vi "Load cell setup.vi"(8 "error in (no error)":errorcluster) -> (0 "error out":errorcluster)   [LabVIEW 2016]
uses:
  Controls/Gain modes.ctl
  <vilib>/Utility/inputDevices.llb/keyboardAcquire.vi
  <vilib>/Utility/inputDevices.llb/closeKeyboard.vi
panel:
  in  "Offset":dbl
  in  "Gain":dbl=1.0
  in  "Confirm":bool
  in  "Cancel":bool
  # "TEST SETTINGS"
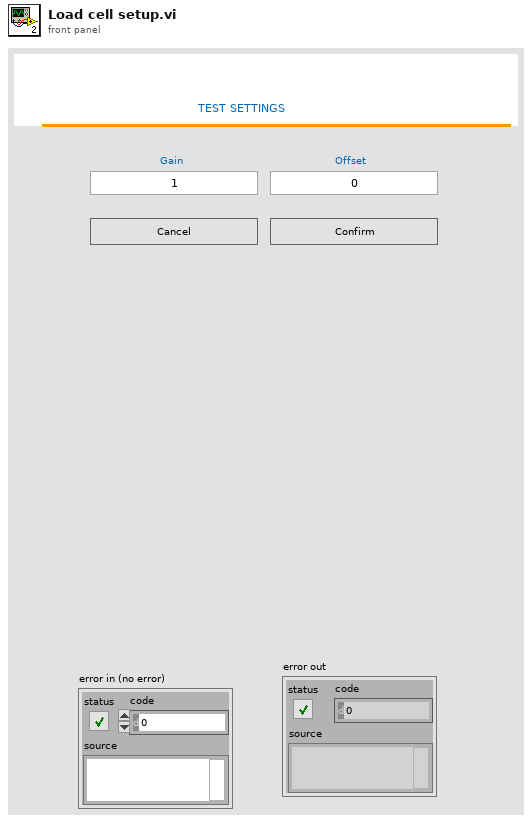
[diagram p1: front panel]
types:
  T1 = typedef "Gain modes.ctl" = enum16{"Initalise", "Get", "Set"}
  T2 = enum16{"0", "1", "2", "3", "4", "5", "6", "7", "8", "9", "A", "B", "C", "D", "E", "F", "G", "H", "I", "J", "K", "L", "M", "N", "O", "P", "Q", "R", "S", "T", "U", "V", "W", "X", "Y", "Z", "F1", "F2", "F3", "F4", "F5", "F6", "F7", "F8", "F9", "F10", "F11", "F12", "F13", "F14", "F15", "ADD", "BACK", "BACKSLASH", "CAPITAL", "COMMA", "DECIMAL", "DELETE", "DIVIDE", "DOWN", "END", "EQUALS", "ESCAPE", "GRAVE (`)", "HOME", "INSERT", "LBRACKET", "LCONTROL", "LEFT", "L ALT", "LSHIFT", "LWIN", "MINUS", "MULTIPLY", "NEXT", "NUMLOCK", "NUMPAD_0", "NUMPAD_1", "NUMPAD_2", "NUMPAD_3", "NUMPAD_4", "NUMPAD_5", "NUMPAD_6", "NUMPAD_7", "NUMPAD_8", "NUMPAD_9", "PAUSE", "PERIOD", "PRIOR (PG UP)", "RBRACKET", "RCONTROL", "RETURN", "RIGHT", "R ALT", "RSHIFT", "RWIN", "SCROLL", "SEMICOLON", "SLASH", "SPACE", "SUBTRACT", "TAB", "UP", "ENTER (num pad)", "' (quote)"}
  T3 = enum16{"0", "1", "2", "3", "4", "5", "6", "7", "8", "9", "A", "B", "C", "D", "E", "F", "G", "H", "I", "J", "K", "L", "M", "N", "O", "P", "Q", "R", "S", "T", "U", "V", "W", "X", "Y", "Z", "F1", "F2", "F3", "F4", "F5", "F6", "F7", "F8", "F9", "F10", "F11", "F12", "F13", "F14", "F15", "ADD", "BACK", "BACKSLASH", "CAPITAL", "COMMA", "DECIMAL", "DELETE", "DIVIDE", "DOWN", "END", "EQUALS", "ESCAPE", "GRAVE (`)", "HOME", "INSERT", "LBRACKET", "LCONTROL", "LEFT", "L ALT", "LSHIFT", "LWIN", "MINUS", "MULTIPLY", "NEXT", "NUMLOCK", "NUMPAD_0", "NUMPAD_1", "NUMPAD_2", "NUMPAD_3", "NUMPAD_4", "NUMPAD_5", "NUMPAD_6", "NUMPAD_7", "NUMPAD_8", "NUMPAD_9", "PAUSE", "PERIOD", "PRIOR (PG UP)", "RBRACKET", "RCONTROL", "RETURN", "RIGHT", "R ALT", "RSHIFT", "RWIN", "SCROLL", "SEMICOLON", "SLASH", "SPACE", "SUBTRACT", "TAB", "UP", "ENTER (num pad)", "' (quote)"}[]
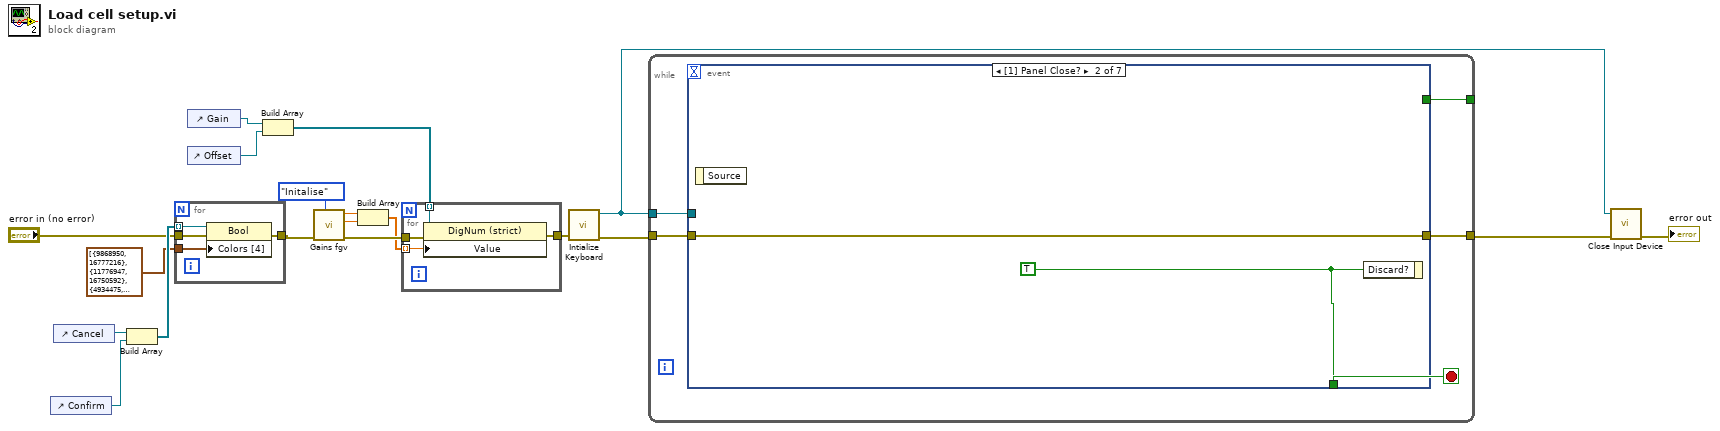
[diagram p0: block diagram]
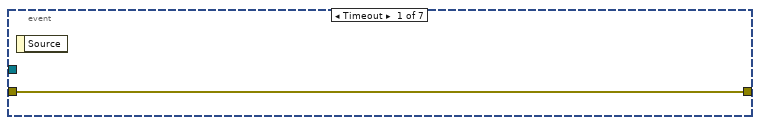
[diagram p2: hidden frame]
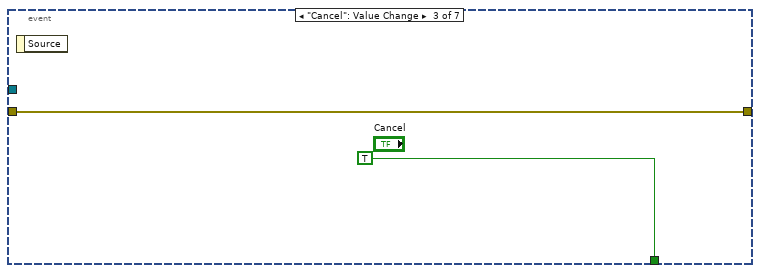
[diagram p3: hidden frame]
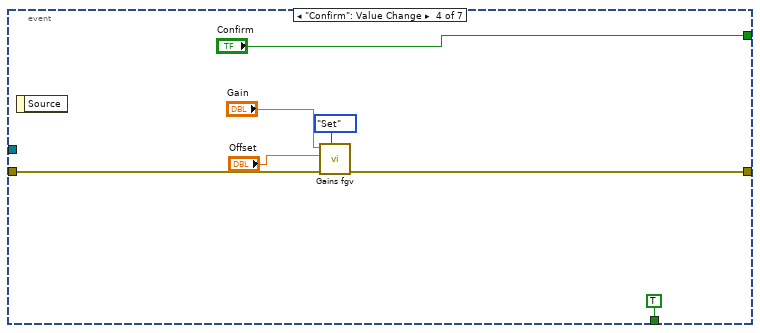
[diagram p4: hidden frame]
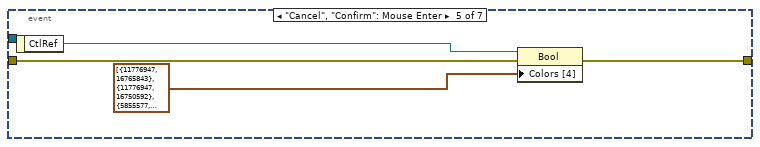
[diagram p5: hidden frame]
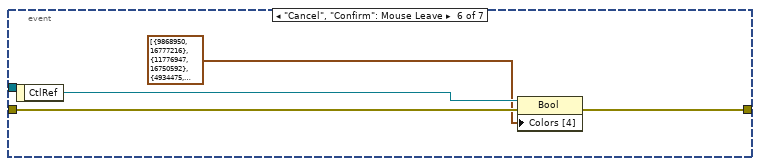
[diagram p6: hidden frame]
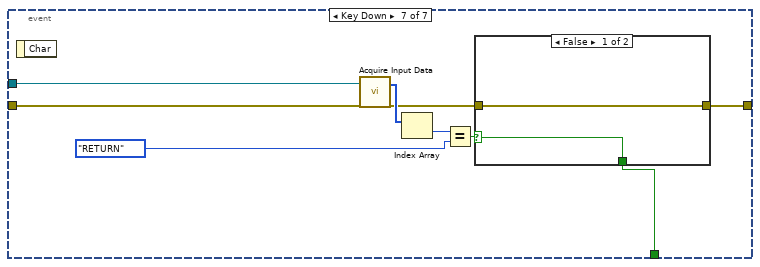
[diagram p7: hidden frame]
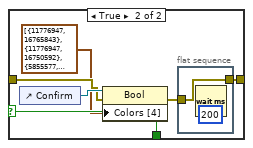
[diagram p8: hidden frame]
diagram:
  n1 = control-ref of="Confirm"() -> (w18:refnum<vi>)
  n2 = control-ref of="Cancel"() -> (w19:refnum<vi>)
  n3 = Build Array(w19, w18) -> (w17:refnum<vi>[])
  n4 = for {
    tunnel: "error in (no error)" -> [w23]
    tunnel: [w22] -> w10
    tunnel: w17 -> [w21] mode=indexing
    tunnel: cluster{u32, u32}[] [{9868950, 16777216}, {11776947, 16750592}, {4934475, 16777216}, {5855577, 8342528}] ("Colors [4]") -> [w20]
    n5 = property class="Bool"(reference=w21, error in=w23, "Colors [4]"=w20) -> (error out=w22:errorcluster)  [unwired: 1 out]
  }
  n6 = control-ref of="Gain"() -> (w4:refnum<vi>)
  n7 = control-ref of="Offset"() -> (w3:refnum<vi>)
  n8 = Build Array(w4, w3) -> (w1:refnum<vi>[])
  n9 = call "Gains fgv.vi"("Mode"=Gain_modes."Initalise", "error in (no error)"=w10) -> ("error out"=w8:errorcluster, "Offset"=w6:dbl, "Gain"=w7:dbl)  [unwired: 7 in]
  n10 = Build Array(w7, w6) -> (w5:dbl[])
  n11 = for {
    tunnel: w8 -> [w27]
    tunnel: w5 -> [w26] mode=indexing
    tunnel: w1 -> [w25] mode=indexing
    tunnel: [w24] -> w2
    n12 = property class="DigNum (strict)"(reference=w25, error in=w27, "Value"=w26) -> (error out=w24:errorcluster)  [unwired: 1 out]
  }
  n13 = call <vilib>:"Intialize Keyboard.vi"("error in (no error)"=w2) -> ("error out"=w15:errorcluster, "device ID"=w12:refnum<k1>)  [unwired: 9 in]
  n14 = while {
    tunnel: w15 -> [w31]
    tunnel: [w30] -> w13
    tunnel: w12 -> [w29]
    tunnel: [w28] -> _
    stop <- w32 stop-if-true
    n15 = event shown="[1] Panel Close?" {
      selector: _ -> [_ _ _ _ _ _ _]
      dyn-events: _ -> [_ _ _ _ _ _ _]
      timeout: _ -> [_ _ _ _ _ _ _]
      tunnel: [_ w35 TRUE ("Discard?") TRUE ("Discard?") _ _ w55] -> w32
      tunnel: w31 -> [w33 w34 w36 w43 w47 w52 w61]
      tunnel: [w33 w34 w36 w39 w46 w51 w53] -> w30
      tunnel: w29 -> [_ _ _ _ _ _ w60]
      tunnel: [_ _ _ "Confirm" _ _ _] -> w28
      event Timeout {
        n16 = event-data() -> ()  [unwired: 1 in, 1 out]
      }
      event Panel Close? {
        w35 = TRUE ("Discard?")
        n17 = event-data() -> ()  [unwired: 1 in, 1 out]
        n18 = event-data("Discard?"=w35) -> ()  [unwired: 1 in, 1 out]
      }
      event "Cancel": Value Change {
        n19 = event-data() -> ()  [unwired: 1 in, 1 out]
      }
      event "Confirm": Value Change {
        n20 = event-data() -> ()  [unwired: 1 in, 1 out]
        n21 = call "Gains fgv.vi"("Mode"=Gain_modes."Set", "error in (no error)"=w43, "Offset"="Offset", "Gain"="Gain") -> ("error out"=w39:errorcluster)  [unwired: 5 in, 2 out]
      }
      event "Cancel", "Confirm": Mouse Enter {
        n22 = event-data() -> ("CtlRef"=w45:refnum<vi>)  [unwired: 1 in]
        n23 = property class="Bool"(reference=w45, error in=w47, "Colors [4]"=cluster{u32, u32}[] [{11776947, 16765843}, {11776947, 16750592}, {5855577, 8350025}, {5855577, 8342528}]) -> (error out=w46:errorcluster)  [unwired: 1 out]
      }
      event "Cancel", "Confirm": Mouse Leave {
        n24 = event-data() -> ("CtlRef"=w50:refnum<vi>)  [unwired: 1 in]
        n25 = property class="Bool"(reference=w50, error in=w52, "Colors [4]"=cluster{u32, u32}[] [{9868950, 16777216}, {11776947, 16750592}, {4934475, 16777216}, {5855577, 8342528}]) -> (error out=w51:errorcluster)  [unwired: 1 out]
      }
      event Key Down {
        n26 = event-data() -> ()  [unwired: 1 in, 1 out]
        n27 = call-poly <vilib>:"Acquire Input Data.vi"("device ID"=w60, "error in (no error)"=w61) -> ("keys pressed"=w59:T3, "error out"=w54:errorcluster)  [unwired: 15 in, 1 out]
        n28 = Index Array(array=w59) -> (element=w58:T2)  [unwired: 1 in]
        n29 = Equal?(x=w58, y=T2."RETURN" ("keyType 3")) -> (x = y?=w56:bool)
        n30 = case shown="False" w56 {
          selector: w56 -> [w62 w69]
          tunnel: [w62 w69] -> w55
          tunnel: w54 -> [w63 w67]
          tunnel: [w63 w64] -> w53
          frame False {
          }
          frame True {
            n31 = control-ref of="Confirm"() -> (w68:refnum<vi>)
            n32 = property class="Bool"(reference=w68, error in=w67, "Colors [4]"=cluster{u32, u32}[] [{11776947, 16765843}, {11776947, 16750592}, {5855577, 8350025}, {5855577, 8342528}]) -> (error out=w65:errorcluster)  [unwired: 1 out]
            n33 = flat-sequence {
              tunnel: w65 -> [w70]
              tunnel: [w70] -> w64
              frame #0 {
                n34 = Wait (ms)(milliseconds to wait=u32 200) -> ()  [unwired: 1 out]
              }
            }
          }
        }
      }
    }
  }
  n35 = call-poly <vilib>:"Close Input Device.vi"("error in (no error)"=w13, "device ID"=w12) -> ("error out"=→"error out":errorcluster)  [unwired: 8 in]
